vi "Generate Hash.vi"(11 "Size (16)":i32=16) -> (2 "Hash Bytes":u8[](array[numeric]), 3 "Hash":string)   [LabVIEW 2017, in "Tree API.lvlib" / "Tree.lvclass"]
doc: "Generate an alphanumeric hash string with size specified in bytes. Not required to be used by the Tree API but can be useful in many other applications. Used internally by the Tree API."
uses:
  Tree.lvclass
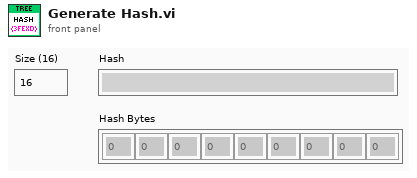
[diagram p1: front panel]
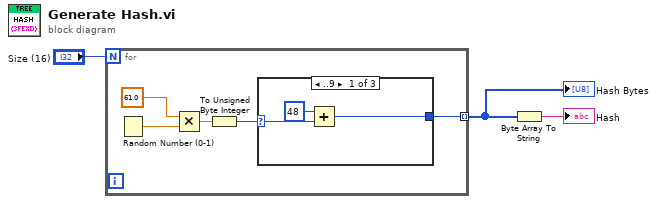
[diagram p0: block diagram]
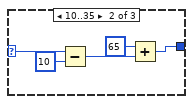
[diagram p2: hidden frame]
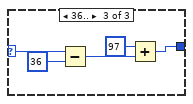
[diagram p3: hidden frame]
diagram:
  n1 = for {
    N: "Size (16)" -> [_]
    tunnel: [w7] -> w1 mode=indexing
    n2 = Random Number (0-1)() -> (number: 0 to 1=w5:dbl)
    n3 = Multiply(x=61.0, y=w5) -> (x*y=w4:dbl)
    n4 = To Unsigned Byte Integer(number=w4) -> (unsigned 8bit integer=w6:u8)
    n5 = case shown="..9" w6 {
      selector: w6 -> [w11 w15 w21]
      tunnel: [w9 w14 w19] -> w7
      frame ..9 {
        n6 = Add(x=u8 48, y=w11) -> (x+y=w9:u8)
      }
      frame 10..35 {
        n7 = Subtract(x=w15, y=u8 10) -> (x-y=w13:u8)
        n8 = Add(x=u8 65, y=w13) -> (x+y=w14:u8)
      }
      frame 36.. {
        n9 = Subtract(x=w21, y=u8 36) -> (x-y=w18:u8)
        n10 = Add(x=u8 97, y=w18) -> (x+y=w19:u8)
      }
    }
  }
  "Hash Bytes" <- w1
  n11 = Byte Array To String(unsigned byte array=w1) -> (string=→"Hash":string)
